vi "Loop_ACT_Right_Motor.vi"() -> ()   [LabVIEW 2017, in "Claw.lvlib"]
uses:
  Claw.lvlib
  _SHARE ALL/TypeDef Share All/CLUSTER_TalonOutput.ctl
  _SHARE ALL/TypeDef Share All/CLUSTER_TalonInput.ctl
  System Drivers/Phoenix-LabVIEW/Motor Controller/Controls/CTRE_Phoenix_MotorControl_ControlMode.ctl
  TypeDef/CLUSTER_PID.ctl
  _SHARE ALL/TypeDef Share All/CONTROL_PositonGraph.ctl
  Globals/Global_Device_IDs.vi
  _SHARE ALL/Global Share All/Global_STOP.vi
  Global_SM Write_Data Out.vi
  System Drivers/Phoenix-LabVIEW/Motor Controller/Get/CTRE_Phoenix_MotorController_GetSelectedSensorData.vi
  System Drivers/Phoenix-LabVIEW/Motor Controller/Get/CTRE_Phoenix_MotorController_GetVoltage.vi
  Global_ACT Write_Data Out.vi
  <vilib>/Rock Robotics/WPI/RobotDrive/WPI_RobotDriveOpen2MotorWithExistingMotors.vi
panel:
  in  "Display Graph":bool
  out "Position Closed Loop Plots":T1
  out "Elbow Input":T2 {"Talon Mode" items=["PercentOutput"=0, "Position"=1, "Velocity"=2, "Current"=3, "Follower"=5, "MotionProfile"=6, "MotionMagic"=7, "MotionMagicArc"=8, "MotionProfileArc"=10, "Disabled"=15]}
  out "Elbow Output":T5
  out "Cycle Time (S)":dbl format="%.3g"
  in  "Target Time(ms)":u32=50
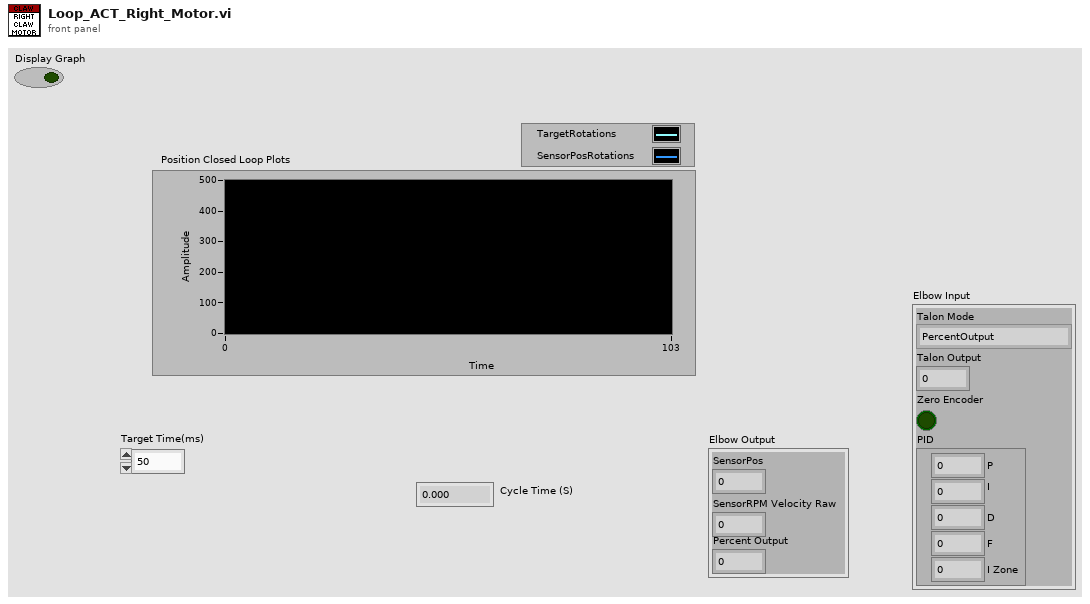
[diagram p1: front panel]
types:
  T1 = typedef "CONTROL_PositonGraph.ctl" = cluster{dbl, "Position (Raw Sensor Units)":i32}
  T2 = typedef "CLUSTER_TalonInput.ctl" = cluster{"Talon Mode":T3, "Talon Output":dbl, "Zero Encoder":bool, "PID":T4}
  T3 = typedef "CTRE_Phoenix_MotorControl_ControlMode.ctl" = u16
  T4 = typedef "CLUSTER_PID.ctl" = cluster{"P":dbl, "I":dbl, "D":dbl, "F":dbl, "I Zone":dbl}
  T5 = typedef "CLUSTER_TalonOutput.ctl" = cluster{"SensorPos":i32, "SensorRPM Velocity Raw":i32, "Percent Output":dbl}
  T6 = typedef "CLUSTER_Claw_Setup.ctl" = cluster{"Left Solenoid":T7, "Right Solenoid":T7, "Left Talon Setup":T9, "Right Talon Setup":T9}
  T7 = typedef "CLUSTER_Solonoid_Setup.ctl" = cluster{"Pneumatics Control Module (0)":u8, "Solenoid Channel":T8}
  T8 = typedef "WPI_SolenoidChannel.ctl" = enum8{"Solenoid 0", "Solenoid 1", "Solenoid 2", "Solenoid 3", "Solenoid 4", "Solenoid 5", "Solenoid 6", "Solenoid 7", "Invalid"}
  T9 = typedef "CLUSTER_Talon_Setup.ctl" = cluster{"Talon SRX ID":u8, "PhaseSensor":bool, "Invert Motor?":bool, "Phoenix Feedback Select":T10, "pidLoopldx":i32, "PID":T4}
  T10 = typedef "CTRE_Phoenix_MotorControl_FeedbackDevice.ctl" = i8
  T11 = typedef "WPI_MotorControlDeviceRef.ctl" = cluster{"DeviceStatus":errorcluster, "Type":T12, "PWM":cluster{"PWM Channel":T13, "DeadBand":T14}, "CAN":cluster{"Device Number":u8, "SetOutput VI Ref":variant, "GetOutput VI Ref":variant, "Enable VI Ref":variant, "Disable VI Ref":variant, "Data":variant}, "Invert":bool, "DIO PWM":cluster{"PWM \"Enable\" Channel":T13, "DIOChannel":T15, "PWM Rate":dbl}}
  T12 = typedef "WPI_MotorControlType.ctl" = enum16{"PWM", "CAN", "DIO PWM"}
  T13 = typedef "FPGA_DIOPWMChannel.ctl" = enum8{"PWM 0", "PWM 1", "PWM 2", "PWM 3", "PWM 4", "PWM 5", "PWM 6", "PWM 7", "PWM 8", "PWM 9", "PWM MXP 0", "PWM MXP 1", "PWM MXP 2", "PWM MXP 3", "PWM MXP 4", "PWM MXP 5", "PWM MXP 6", "PWM MXP 7", "PWM MXP 8", "PWM MXP 9", "Invalid"}
  T14 = typedef "WPI_PWMDeadband.ctl" = cluster{"Name":string, "maxPositivePwm":i32, "minPositivePwm":i32, "centerPwm":i32, "maxNegativePwm":i32, "minNegativePwm":i32, "angularRange":u16}
  T15 = typedef "FPGA_DIOChannel.ctl" = enum8{"DIO 0", "DIO 1", "DIO 2", "DIO 3", "DIO 4", "DIO 5", "DIO 6", "DIO 7", "DIO 8", "DIO 9", "DIO MXP 0", "DIO MXP 1", "DIO MXP 2", "DIO MXP 3", "DIO MXP 4", "DIO MXP 5", "DIO MXP 6", "DIO MXP 7", "DIO MXP 8", "DIO MXP 9", "DIO MXP 10", "DIO MXP 11", "DIO MXP 12", "DIO MXP 13", "DIO MXP 14", "DIO MXP 15", "SPI Port CS1", "SPI Port CS2", "SPI Port CS3", "SPI Port MISO", "SPI Port MOSI", "Invalid"}
  T16 = cluster{"PhoenixMotorControlDevRef":T11, "Left Claw Output":T5, "Left Claw Input":T2, "Target Time(ms)":u32, "Current Time":timestamp, "Previous Time":timestamp, "Cycle Time (S)":dbl, "Last PID":T4}
  T17 = typedef "WPI_RobotDriveDevRef.ctl" = cluster{"DevStatus":errorcluster, "Motors[]":T11[], "Square Inputs":bool, "Max Output":dbl}
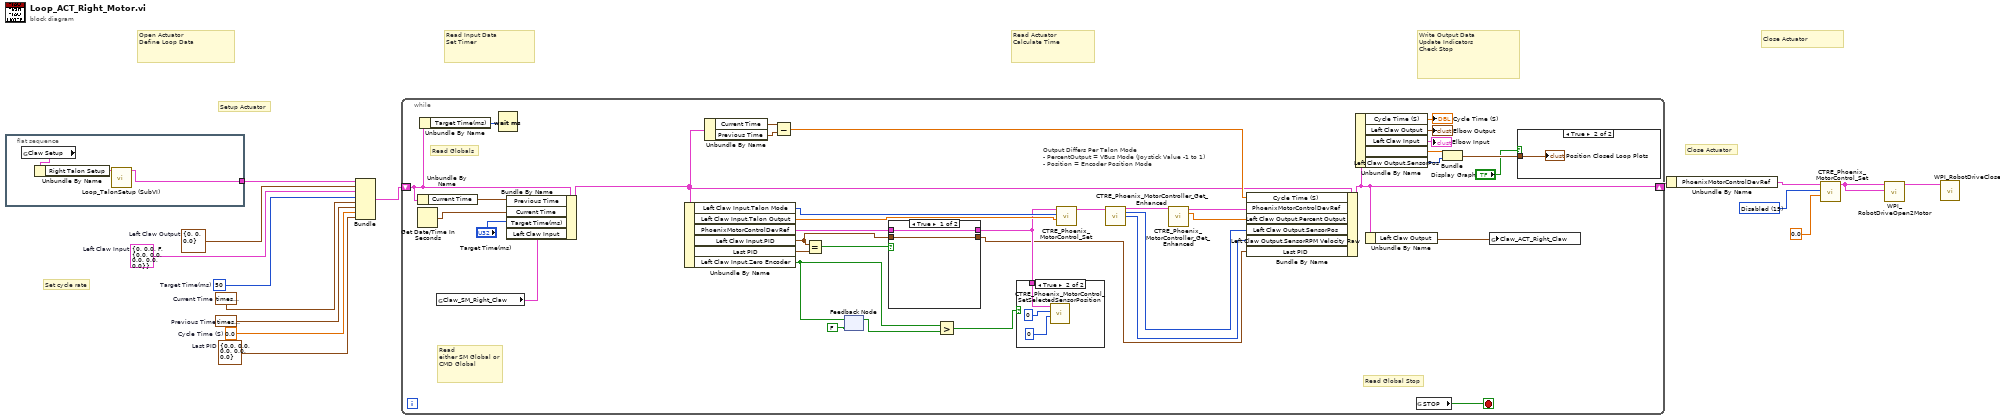
[diagram p0: block diagram]
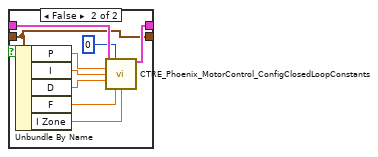
[diagram p2: hidden frame]
diagram:
  w2 = T4 {"P"=0.0, "I"=0.0, "D"=0.0, "F"=0.0, "I Zone"=0.0}  # Last PID
  w6 = T3 15 items=["PercentOutput"=0, "Position"=1, "Velocity"=2, "Current"=3, "Follower"=5, "MotionProfile"=6, "MotionMagic"=7, "MotionMagicArc"=8, "MotionProfileArc"=10, "Disabled"=15] ("Control Mode")
  w8 = T5 {"SensorPos"=0, "SensorRPM Velocity Raw"=0, "Percent Output"=0.0}  # Left Claw Output
  w9 = T2 {"Talon Mode"=0, "Talon Output"=0.0, "Zero Encoder"=FALSE, "PID"={"P"=0.0, "I"=0.0, "D"=0.0, "F"=0.0, "I Zone"=0.0}}  # Left Claw Input
  w10 = 0.0  # Cycle Time (S)
  w15 = timestamp(0 s since 1904-01-01)  # Previous Time
  w14 = timestamp(0 s since 1904-01-01)  # Current Time
  w13 = u32 50  # Target Time(ms)
  # "Close Actuator"
  # "Write Output Data\nUpdate Indicators\nCheck Stop"
  # "Read Actuator\nCalculate Time"
  # "Read Input Data\nSet Timer"
  # "Open Actuator\nDefine Loop Data"
  # "Set cycle rate"
  # "Close Actuator"
  # "Setup Actuator"
  n1 = flat-sequence {
    tunnel: [w17] -> w1
    frame #0 {
      n2 = global read "Global_Device_IDs.vi" "Claw Setup"() -> (w18:T6)
      n3 = Unbundle By Name(w18) -> ("Right Talon Setup"=w16:T9)
      n4 = call "Loop_TalonSetup (SubVI).vi"("Elbow Setup"=w16) -> ("PhoenixMotorControlDevRef"=w17:T11)  [unwired: 10 in]
    }
  }
  n5 = Bundle("PhoenixMotorControlDevRef"=w1, "Left Claw Output"=w8, "Left Claw Input"=w9, "Target Time(ms)"=w13, "Current Time"=w14, "Previous Time"=w15, "Cycle Time (S)"=w10, "Last PID"=w2) -> (w12:T16)  [unwired: 1 in]
  n6 = while {
    shift-right: [w48] -> w11
    shift-left: w12 -> [w50]
    stop <- w56 stop-if-true
    # "Output Differs Per Talon Mode\n- PercentOutput = VBus Mode (Joystick Value -1 to 1)\n- Position = Encoder Position Mode"
    # "Read\neither SM Global or CMD Global"
    # "Read Globals"
    # "Read Global Stop"
    n7 = Unbundle By Name(w50) -> ("Current Time"=w54:timestamp)
    n8 = Get Date/Time In Seconds() -> (seconds since 1Jan1904=w55:timestamp)
    n9 = Unbundle By Name(w50) -> ("Target Time(ms)"=w49:u32)
    n10 = global read "Global_SM Write_Data Out.vi" "Claw_SM_Right_Claw"() -> (w20:T2)
    n11 = Wait (ms)(milliseconds to wait=w49) -> ()  [unwired: 1 out]
    n12 = Bundle By Name(cluster=w50, "Previous Time"=w54, "Current Time"=w55, "Target Time(ms)"="Target Time(ms)", "Left Claw Input"=w20) -> (w33:T16)
    n13 = Unbundle By Name(w33) -> ("Left Claw Input.Talon Mode"=w45:T3, "Left Claw Input.Talon Output"=w44:dbl, "PhoenixMotorControlDevRef"=w32:T11, "Left Claw Input.PID"=w28:T4, "Last PID"=w29:T4, "Left Claw Input.Zero Encoder"=w23:bool)
    n14 = Unbundle By Name(w33) -> ("Current Time"=w53:timestamp, "Previous Time"=w52:timestamp)
    n15 = Subtract(x=w53, y=w52) -> (x-y=w46:dbl)
    n16 = Equal?(x=w28, y=w29) -> (x = y?=w26:bool)
    n17 = feedback #1(FALSE) -> (w24:bool)
    n18 = feedback-in #1(w23) -> ()
    n19 = case shown="True" w26 {
      tunnel: w32 -> [w58 w67]
      tunnel: [w58 w66] -> w31
      tunnel: w28 -> [w57 w59]
      tunnel: [w57 w59] -> w27
      frame True {
      }
      frame False {
        n20 = Unbundle By Name(w59) -> ("P"=w64:dbl, "I"=w63:dbl, "D"=w62:dbl, "F"=w61:dbl, "I Zone"=w60:dbl)
        n21 = call "CTRE_Phoenix_MotorControl_ConfigClosedLoopConstants.vi"("PhoenixMotorControlDevRef"=w67, "slotIdx"=0, "P"=w64, "I"=w63, "D"=w62, "F"=w61, "I Zone"=w60) -> ("PhoenixMotorControlDevRef"=w66:T11)  [unwired: 7 in, 1 out]
      }
    }
    n22 = Greater?(x=w23, y=w24) -> (0:w22:bool)
    n23 = case shown="True" w22 {
      tunnel: w31 -> [_ w71]
      frame False {
      }
      frame True {
        n24 = call "CTRE_Phoenix_MotorControl_SetSelectedSensorPosition.vi"("pidLoopIdx"=u32 0, "New Sensor Position"=0, "PhoenixMotorControlDevRef"=w71) -> ()  [unwired: 7 in, 2 out]
      }
    }
    n25 = call "CTRE_Phoenix_MotorControl_Set.vi"("Output"=w44, "Control Mode"=w45, "PhoenixMotorControlDevRef"=w31) -> ("PhoenixMotorControlDevRef"=w43:T11)  [unwired: 7 in, 1 out]
    n26 = call-poly "CTRE_Phoenix_MotorController_Get_Enhanced.vi"("PhoenixMotorControlDevRef"=w43) -> ("PhoenixMotorControlDevRef"=w42:T11, "Position (Raw Sensor Units)"=w39:i32, "Velocity (Raw Sensor Units per 100 ms)"=w40:i32)  [unwired: 11 in, 1 out]
    n27 = call-poly "CTRE_Phoenix_MotorController_Get_Enhanced.vi"("PhoenixMotorControlDevRef"=w42) -> ("PhoenixMotorControlDevRef"=w21:T11, "Percent Output"=w41:dbl)  [unwired: 10 in, 3 out]
    n28 = Bundle By Name(cluster=w33, "Cycle Time (S)"=w46, "PhoenixMotorControlDevRef"=w21, "Left Claw Output.Percent Output"=w41, "Left Claw Output.SensorPos"=w39, "Left Claw Output.SensorRPM Velocity Raw"=w40, "Last PID"=w27) -> (w48:T16)
    n29 = Unbundle By Name(w48) -> ("Cycle Time (S)"=→"Cycle Time (S)":dbl, "Left Claw Output"=→"Elbow Output":T5, "Left Claw Input"=→"Elbow Input":T2, "Left Claw Input.Talon Output"=w36:dbl, "Left Claw Output.SensorPos"=w35:i32)
    n30 = Unbundle By Name(w48) -> ("Left Claw Output"=w19:T5)
    n31 = global read "Global_STOP.vi" "STOP"() -> (w56:bool)
    n32 = Bundle("Talon Output"=w36, "SensorPos"=w35) -> (w34:cluster{"Talon Output":dbl, "SensorPos":i32})  [unwired: 1 in]
    n33 = global write "Global_ACT Write_Data Out.vi" "Claw_ACT_Right_Claw"(w19) -> ()
    n34 = case shown="True" "Display Graph" {
      tunnel: w34 -> [_ w68]
      frame False {
      }
      frame True {
        "Position Closed Loop Plots" <- w68
      }
    }
  }
  n35 = Unbundle By Name(w11) -> ("PhoenixMotorControlDevRef"=w7:T11)
  n36 = call "CTRE_Phoenix_MotorControl_Set.vi"("Output"=0.0, "Control Mode"=w6, "PhoenixMotorControlDevRef"=w7) -> ("PhoenixMotorControlDevRef"=w3:T11)  [unwired: 7 in, 1 out]
  n37 = call-poly <vilib>:"WPI_RobotDriveOpen2Motor.vi"("Right Motor Dev Ref"=w3, "Left Motor Dev Ref"=w3) -> ("RobotDriveDevRef"=w5:T17)  [unwired: 8 in, 1 out]
  n38 = call <vilib>:"WPI_RobotDriveClose.vi"("RobotDriveDevRef"=w5) -> ()  [unwired: 10 in, 1 out]
